vi "Display Tree Item.vi"(8 "error in (no error)":errorcluster, 10 "Tag":string, 11 "Application Data in":T1) -> (0 "error out":errorcluster, 3 "Application Data out":T1)   [LabVIEW 2017, in "DSF Configuration Utility.lvlib"]
uses:
  DSF Configuration Utility.lvlib
  Application Data.ctl
  DSF Configuration API/1.0.0/Public/Controls/DSF Config Data RefNum.ctl
  View Mode.ctl
  DSF Configuration API/1.0.0/Public/Read Item/Read Plugin.vi
  DSF Configuration API/1.0.0/Public/Read Item/Read Settings.vi
  DSF Configuration API/1.0.0/Public/Read Item/Read Channel.vi
  DSF Configuration API/1.0.0/Public/Read Item/Read Transfer.vi
  DSF Configuration API/1.0.0/Public/Read Item/Read Group.vi
  DSF Configuration API/1.0.0/DSF Configuration API.lvlib
panel:
  # "App\nData"
  # "App\nData"
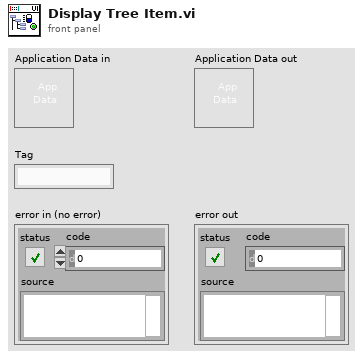
[diagram p1: front panel]
types:
  T1 = typedef "DSF Configuration Utility.lvlib/Application Data.ctl" = cluster{"Item Tree Control":refnum<vi>, "Value Tree Control":refnum<vi>, "DSF Refnum":T2, "Top-Level VI":refnum<vi>, "View State":T3, "menu reference":refnum<k9>}
  T2 = typedef "DSF Configuration API.lvlib/DSF Config Data RefNum.ctl" = refnum<k1>
  T3 = typedef "DSF Configuration Utility.lvlib/View Mode.ctl" = enum16{"Tree", "List"}
  T4 = typedef "DSF Configuration API.lvlib/DSF Version Info.ctl" = cluster{"major":u32, "minor":u32, "fix":u32, "build":string}
  T5 = typedef "DSF Configuration Utility.lvlib/Tree Item Type.ctl" = enum16{"Plugin", "Group", "Transfer", "Channel", "Setting"}
  T6 = typedef "DSF Configuration API.lvlib/DSF Group Info.ctl" = cluster{"direction":T7, "timing":T8, "transfer ids":string[], "settings id":string}
  T7 = typedef "DSF Configuration API.lvlib/DSF Direction.ctl" = enum8{"Tx", "Rx"}
  T8 = typedef "DSF Configuration API.lvlib/DSF Timing Info.ctl" = cluster{"priority":i32, "decimation":i32, "offset":i32}
  T9 = typedef "DSF Configuration API.lvlib/DSF Transfer Info.ctl" = cluster{"byte order":T10, "channel ids":string[], "settings id":string}
  T10 = typedef "DSF Configuration API.lvlib/DSF Byte Order.ctl" = enum8{"big-endian", "little-endian"}
  T11 = typedef "DSF Configuration API.lvlib/DSF Channel Info.ctl" = cluster{"count":i32, "offset":i32, "data type":T12, "resource path":string, "settings id":string}
  T12 = typedef "DSF Configuration API.lvlib/DSF Data Type.ctl" = enum8{"Bool", "SGL", "DBL", "I8", "I16", "I32", "I64", "U8", "U16", "U32", "U64"}
  T13 = typedef "DSF Configuration API.lvlib/DSF Settings Info.ctl" = cluster{"key":string, "value":string}[]
  T14 = typedef "DSF Configuration API.lvlib/DSF Plugin Info.ctl" = cluster{"type":string, "timing":T8, "group ids":string[], "settings id":string}
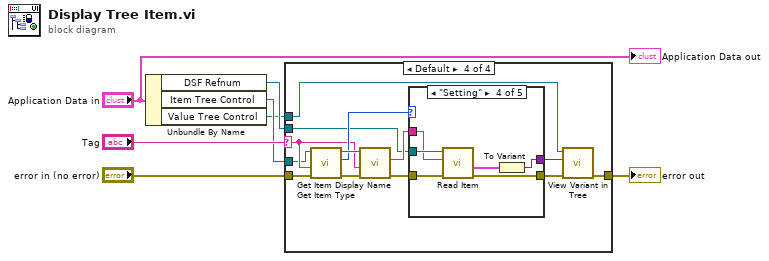
[diagram p0: block diagram]
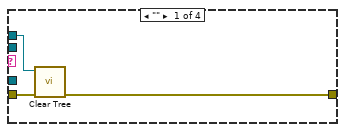
[diagram p2: hidden frame]
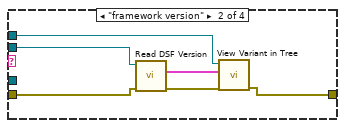
[diagram p3: hidden frame]
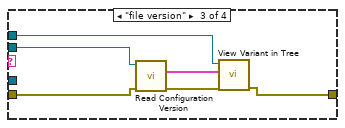
[diagram p4: hidden frame]
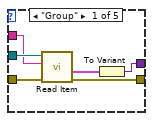
[diagram p5: hidden frame]
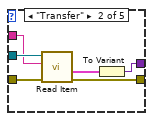
[diagram p6: hidden frame]
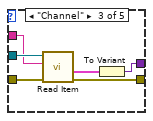
[diagram p7: hidden frame]
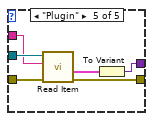
[diagram p8: hidden frame]
diagram:
  n1 = Unbundle By Name("Application Data in") -> ("DSF Refnum"=w5:T2, "Item Tree Control"=w4:refnum<vi>, "Value Tree Control"=w2:refnum<vi>)
  n2 = case shown="Default" "Tag" {
    selector: "Tag" -> [_ _ _ w30]
    tunnel: w5 -> [_ w16 w22 w29]
    tunnel: w4 -> [_ _ _ w28]
    tunnel: "error in (no error)" -> [w10 w15 w21 w27]
    tunnel: w2 -> [w8 w11 w17 w24]
    tunnel: [w9 w13 w19 w23] -> w1
    frame "" {
      n3 = call "Clear Tree.vi"("error in (no error)"=w10, "TreeControl in"=w8) -> ("error out"=w9:errorcluster)  [unwired: 9 in]
    }
    frame "framework version" {
      n4 = call "Read DSF Version.vi"("error in (no error)"=w15, "dsf refnum"=w16) -> ("error out"=w14:errorcluster, "dsfversion"=w12:T4)  [unwired: 7 in, 1 out]
      n5 = call "View Variant in Tree.vi"("error in (no error)"=w14, "Variant"=w12, "TreeControl in"=w11) -> ("error out"=w13:errorcluster)  [unwired: 8 in]
    }
    frame "file version" {
      n6 = call "Read Configuration Version.vi"("error in (no error)"=w21, "dsf refnum"=w22) -> ("error out"=w20:errorcluster, "version"=w18:T4)  [unwired: 7 in, 1 out]
      n7 = call "View Variant in Tree.vi"("error in (no error)"=w20, "Variant"=w18, "TreeControl in"=w17) -> ("error out"=w19:errorcluster)  [unwired: 8 in]
    }
    frame Default {
      n8 = call "Get Item Type.vi"("error in (no error)"=w27, "Tag"=w30, "TreeControl in"=w28) -> ("error out"=w34:errorcluster, "Item Type"=w32:T5, "TreeControl out"=w33:refnum<vi>)  [unwired: 6 in]
      n9 = call "Get Item Display Name.vi"("error in (no error)"=w34, "Tag"=w30, "TreeControl in"=w33) -> ("error out"=w35:errorcluster, "display name"=w31:string)  [unwired: 6 in, 1 out]
      n10 = case shown="\"Setting\"" w32 {
        tunnel: w31 -> [w36 w42 w48 w54 w60]
        tunnel: [w40 w45 w51 w58 w64] -> w26
        tunnel: w35 -> [w39 w46 w52 w59 w65]
        tunnel: w29 -> [w38 w44 w50 w57 w63]
        tunnel: [w37 w43 w49 w55 w62] -> w25
        frame "Group" {
          n11 = call-poly "Read Item.vi"("error in (no error)"=w39, "name"=w36, "dsf refnum"=w38) -> ("error out"=w40:errorcluster, "value"=w41:T6)  [unwired: 5 in, 2 out]
          n12 = To Variant(anything=w41) -> (Variant=w37:variant)
        }
        frame "Transfer" {
          n13 = call-poly "Read Item.vi"("error in (no error)"=w46, "name"=w42, "dsf refnum"=w44) -> ("error out"=w45:errorcluster, "value"=w47:T9)  [unwired: 5 in, 2 out]
          n14 = To Variant(anything=w47) -> (Variant=w43:variant)
        }
        frame "Channel" {
          n15 = call-poly "Read Item.vi"("error in (no error)"=w52, "name"=w48, "dsf refnum"=w50) -> ("error out"=w51:errorcluster, "value"=w53:T11)  [unwired: 5 in, 2 out]
          n16 = To Variant(anything=w53) -> (Variant=w49:variant)
        }
        frame "Setting" {
          n17 = call-poly "Read Item.vi"("error in (no error)"=w59, "name"=w54, "dsf refnum"=w57) -> ("error out"=w58:errorcluster, "value"=w56:T13)  [unwired: 5 in, 2 out]
          n18 = To Variant(anything=w56) -> (Variant=w55:variant)
        }
        frame "Plugin" {
          n19 = call-poly "Read Item.vi"("error in (no error)"=w65, "name"=w60, "dsf refnum"=w63) -> ("error out"=w64:errorcluster, "value"=w61:T14)  [unwired: 5 in, 2 out]
          n20 = To Variant(anything=w61) -> (Variant=w62:variant)
        }
      }
      n21 = call "View Variant in Tree.vi"("error in (no error)"=w26, "Variant"=w25, "TreeControl in"=w24) -> ("error out"=w23:errorcluster)  [unwired: 8 in]
    }
  }
  "error out" <- w1
  "Application Data out" <- "Application Data in"
